vi "PC Main.vi"() -> ()   [LabVIEW 2021]
uses:
  Type Definitions/Computer Metadata.ctl
  Type Definitions/Internet Connection Monitor.ctl
  Type Definitions/CPU Usage.ctl
  Type Definitions/Disk State.ctl
  Type Definitions/Memory Monitor.ctl
  Type Definitions/System Time.ctl
  Type Definitions/Payload Class.ctl
  Type Definitions/Data Frame Header.ctl
  Type Definitions/Data Frame.ctl
  Type Definitions/Telemetry TCP State.ctl
  Type Definitions/Telemetry Recorder Status.ctl
  Type Definitions/Queue Monitor.ctl
  Type Definitions/RTOSMonitor.ctl
  Type Definitions/Enum - Commands.ctl
  Type Definitions/Command TCP State.ctl
  Type Definitions/Enum - Notification Types.ctl
  Type Definitions/Notification Data.ctl
  Type Definitions/Network Adapter State.ctl
  Type Definitions/Discovery Engine State.ctl
  Type Definitions/Digital Output Data.ctl
  Type Definitions/Analog Output Data.ctl
  <vilib>/ptbypt/NI_PtbyPt.lvlib
  Type Definitions/Computer Resources.ctl
  Type Definitions/RT Image Metadata.ctl
  Type Definitions/Startup Settings.ctl
  Type Definitions/Digital Input Data.ctl
  Type Definitions/Writeable Drives.ctl
  Type Definitions/Analog Data.ctl
  Type Definitions/GPS Solution Data.ctl
  Type Definitions/Device.ctl
  <vilib>/Utility/tcp.llb/UDP Multicast Read-Only Open.vi
  Type Definitions/Analog Output Command.ctl
  Type Definitions/Digital Output Command.ctl
panel:
  in  "Source to View":T1
  out "Data Rate (Mbps)":dbl
  out "Telemetry Rate (Packets/s)":i32
  out "Telemetry IP Address":string
  out "Detected IP Addresses":string[](array[string])
  out "Valid IP Addresses":i32
  out "Telemetry Handler":T2 {"CRC" format="%08x"; "Frame Header"."Options" format="%016b"; "Frame Header"."Time" format="%^<%I:%M:%S%3u %p\n%m/%d/%Y %Z>T"; "Frame Header"."Sync" format="%08x"}
  in  "Main Tabs":T5(tab)
  out "Computer Metadata":T6
  out "Computer Resources":T7
  out "RT Image Metadata":T8
  out "Startup Settings":T9
  out "CPU Utilization":dbl[][](graph)
  out "Available Memory":dbl[][](graph)
  out "Internet Connection Monitor":T10
  out "CPU Monitor":T11 {"Idle CPU Time" format="%#.2f"; "SIRQ CPU Usage" format="%#.2f"; "IRQ CPU Usage" format="%#.2f"; "IO CPU Usage" format="%#.2f"; "NIC CPU" format="%#.2f"; "System CPU Usage" format="%#.2f"; "User CPU Usage" format="%#.2f"}
  out "Memory Monitor":T12 {"Available Memory" format="%#.2f"; "Total Memory" format="%#.2f"}
  out "RTOS Monitor":T13[](array[typedef])
  out "Archive Monitor":T14
  out "Queue Monitor":T15[](array[typedef])
  out "System Time":T16 {"GPS Clock" format="%^<%I:%M:%S%3u %p\n%m/%d/%Y %Z>T"; "System Clock" format="%^<%I:%M:%S%3u %p\n%m/%d/%Y %Z>T"}
  out "Telemetry TCP State":T17
  out "Command TCP State":T18
  out "Network Adapter State":T19
  out "Discovery Engine State":T20[](array[typedef])
  out "Disk Management":T21[](array[typedef]) {"Used" format="%#.2f"; "Available" format="%#.2f"; "Total" format="%#.2f"}
  out "Writeable Drives":T22
  out "Digital Input Data":i16[][](graph)
  out "Analog Output Data":dbl[][](graph)
  out "Analog Input Data":sgl[][](graph)
  out "Notification Data":cluster{"Time":dbl, T23} {"Time" format="%^<%I:%M:%S%3u %p\n%m/%d/%Y %Z>T"}
  out "GPS Solution Data":T25 {"GPS Timestamp" format="%^<%I:%M:%S%3u %p\n%m/%d/%Y %Z>T"}
  in  "Send Digital Command":bool
  in  "Digital Output Command":T26
  in  "Null Command":bool
  out "Command Ack":T2 {"CRC" format="%08x"; "Frame Header"."Options" format="%016b"; "Frame Header"."Time" format="%^<%I:%M:%S%3u %p\n%m/%d/%Y %Z>T"; "Frame Header"."Sync" format="%08x"}
  out "Digital Output Data":T27 {"Port 0" format="%08b"}
  in  "Send Analog Command":bool
  in  "Analog Output Command":T28 {"State" scale=0.0..5.0}
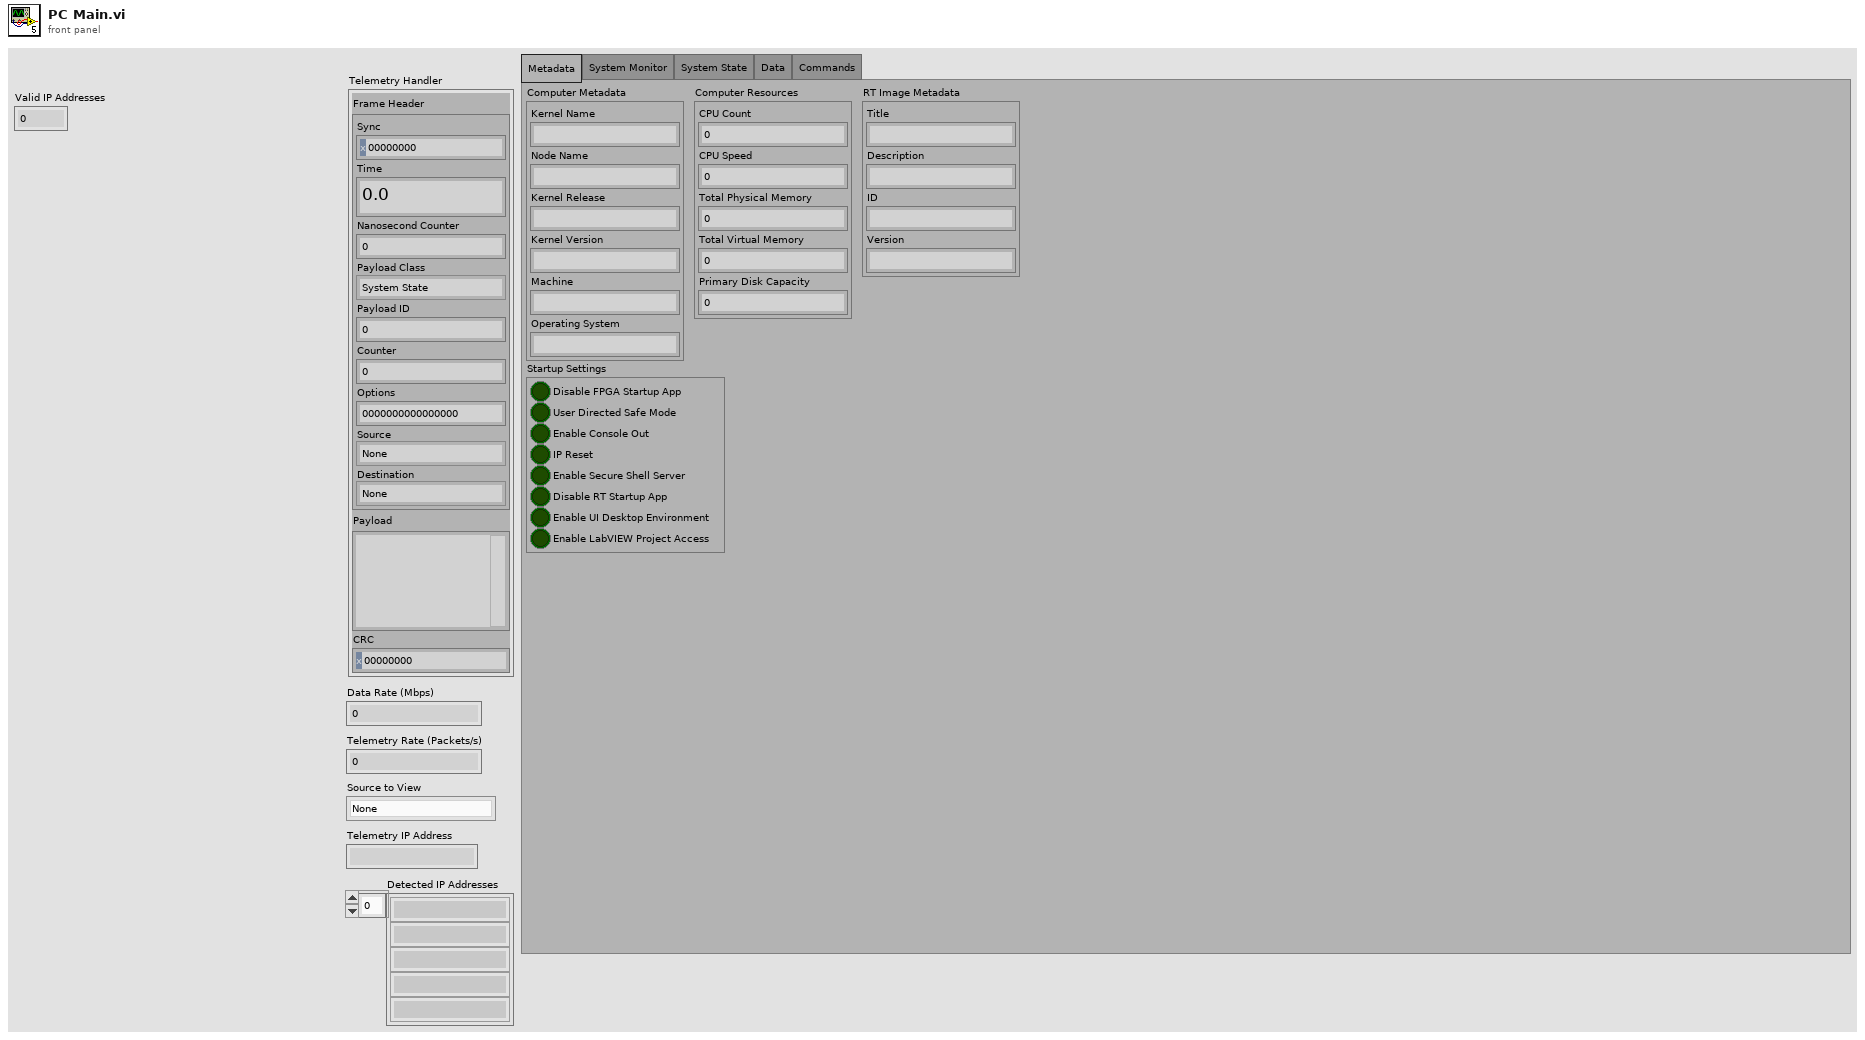
[diagram p1: front panel]
types:
  T1 = typedef "Device.ctl" = enum32{"None", "Exec", "Aux1", "Aux2", "Aux3"}
  T2 = typedef "Data Frame.ctl" = cluster{"Frame Header":T3, "Payload":string, "CRC":u32}
  T3 = typedef "Data Frame Header.ctl" = cluster{"Sync":u32, "Time":dbl, "Nanosecond Counter":i64, "Payload Class":T4, "Payload ID":u16, "Counter":i32, "Options":u32, "Source":T1, "Destination":T1}
  T4 = typedef "Payload Class.ctl" = enum16{"System State", "Parameters", "Metadata", "Software Monitor", "Data", "Commands"}
  T5 = enum32{"Metadata", "System Monitor", "System State", "Data", "Commands"}
  T6 = typedef "Computer Metadata.ctl" = cluster{"Kernel Name":string, "Node Name":string, "Kernel Release":string, "Kernel Version":string, "Machine":string, "Operating System":string}
  T7 = typedef "Computer Resources.ctl" = cluster{"CPU Count":i32, "CPU Speed":u32, "Total Physical Memory":dbl, "Total Virtual Memory":dbl, "Primary Disk Capacity":dbl}
  T8 = typedef "RT Image Metadata.ctl" = cluster{"Title":string, "Description":string, "ID":string, "Version":string}
  T9 = typedef "Startup Settings.ctl" = cluster{"Disable FPGA Startup App":bool, "User Directed Safe Mode":bool, "Enable Console Out":bool, "IP Reset":bool, "Enable Secure Shell Server":bool, "Disable RT Startup App":bool, "Enable UI Desktop Environment":bool, "Enable LabVIEW Project Access":bool}
  T10 = typedef "Internet Connection Monitor.ctl" = cluster{"Connected?":bool, "Ping Latency (uS)":i32, "Ping Address":string}
  T11 = typedef "CPU Usage.ctl" = cluster{"User CPU Usage":sgl, "System CPU Usage":sgl, "NIC CPU ":sgl, "IO CPU Usage":sgl, "IRQ CPU Usage":sgl, "SIRQ CPU Usage":sgl, "Idle CPU Time":sgl}
  T12 = typedef "Memory Monitor.ctl" = cluster{"Total Memory":sgl, "Available Memory":sgl}
  T13 = typedef "RTOSMonitor.ctl" = cluster{"Task Name":string, "Priority":i32, "Processor":i32, "Offset":i64, "Min Duration":i64, "Mean Duration":i64, "Max Duration":i64, "Period":i64, "Late Iterations":i16, "Iteration Count":i32}
  T14 = typedef "Telemetry Recorder Status.ctl" = cluster{"Filepath":string, "File Size":i64, "Frame Count":i32, "Mean MB/hour":sgl}
  T15 = typedef "Queue Monitor.ctl" = cluster{"Queue Name":string, "Max Queue Size":i32, "Pending Remove":i32, "Pending Insert":i32, "Elements in Queue":i32}
  T16 = typedef "System Time.ctl" = cluster{"System Clock":timestamp, "GPS Clock":timestamp, "Nanosecond Counter":i64, "GPS Status":enum8{"Initializing", "Normal", "Unable to get fix"}, "GPS Antenna Status":enum8{"Unknown", "Normal", "Absent", "Overcurrent"}, "GPS Satelites Available":u8, "GPS Time (ns)":u64, "GPS UTC Offset":i8, "GPS Time Offset":i32, "UTC Offset Valid":bool, "GPS Time Lock":bool}
  T17 = typedef "Telemetry TCP State.ctl" = cluster{"Is Connected":bool, "Remote Address":string, "Remote Port":u16, "Total Frames Sent":i32, "Total Bytes Sent":i32}
  T18 = typedef "Command TCP State.ctl" = cluster{"Is Connected":bool, "Remote Address":string, "Remote Port":u16, "Total Frames Sent":i32, "Total Bytes Sent":i32}
  T19 = typedef "Network Adapter State.ctl" = cluster{"Adapter IP Addresses":string[]}
  T20 = typedef "Discovery Engine State.ctl" = cluster{"Adapter IP Address":string, "Connection ID":refnum<k16>, "Error":errorcluster}
  T21 = typedef "Disk State.ctl" = cluster{"File System Name":string, "Total":sgl, "Available":sgl, "Used":sgl, "Path":string}
  T22 = typedef "Writeable Drives.ctl" = cluster{"USB/SD Drives":path[], "Hard Drives":path[]}
  T23 = typedef "Notification Data.ctl" = cluster{"Notification Type":T24, "Code":i32, "Description":string}
  T24 = typedef "Enum - Notification Types.ctl" = enum16{"Warning", "Acknowledge", "Notification"}
  T25 = typedef "GPS Solution Data.ctl" = cluster{"GPS Timestamp":timestamp, "GPS Status":enum8{"Initializing", "Normal", "Unable to get fix"}, "GPS Antenna Status":enum8{"Unknown", "Normal", "Absent", "Overcurrent"}, "GPS Satelites Available":u8, "GPS Time Lock":bool, "GPS UTC Offset Valid":bool, "GPS Self-Survey Complete":bool, "GPS Latitude (°)":dbl, "GPS Longitude (°)":dbl, "GPS Altitude (m)":dbl, "GPS Serial Number":u32, "GPS Vendor ID":u16, "GPS Firmware Version":u32}
  T26 = typedef "Digital Output Command.ctl" = cluster{"DO Channel":u8, "State":bool}
  T27 = typedef "Digital Output Data.ctl" = cluster{"Port 0":u8}
  T28 = typedef "Analog Output Command.ctl" = cluster{"AO Channel":u8, "State":dbl}
  T29 = typedef "Enum - Commands.ctl" = enum16{"Null", "Analog Output Command", "Digital Output Command"}
  T30 = typedef "Analog Data.ctl" = cluster{"Analog Data":sgl[][]}
  T31 = typedef "Analog Output Data.ctl" = cluster{"Bank 0":dbl[]}
  T32 = typedef "Digital Input Data.ctl" = cluster{"Digital Data":u64[][]}
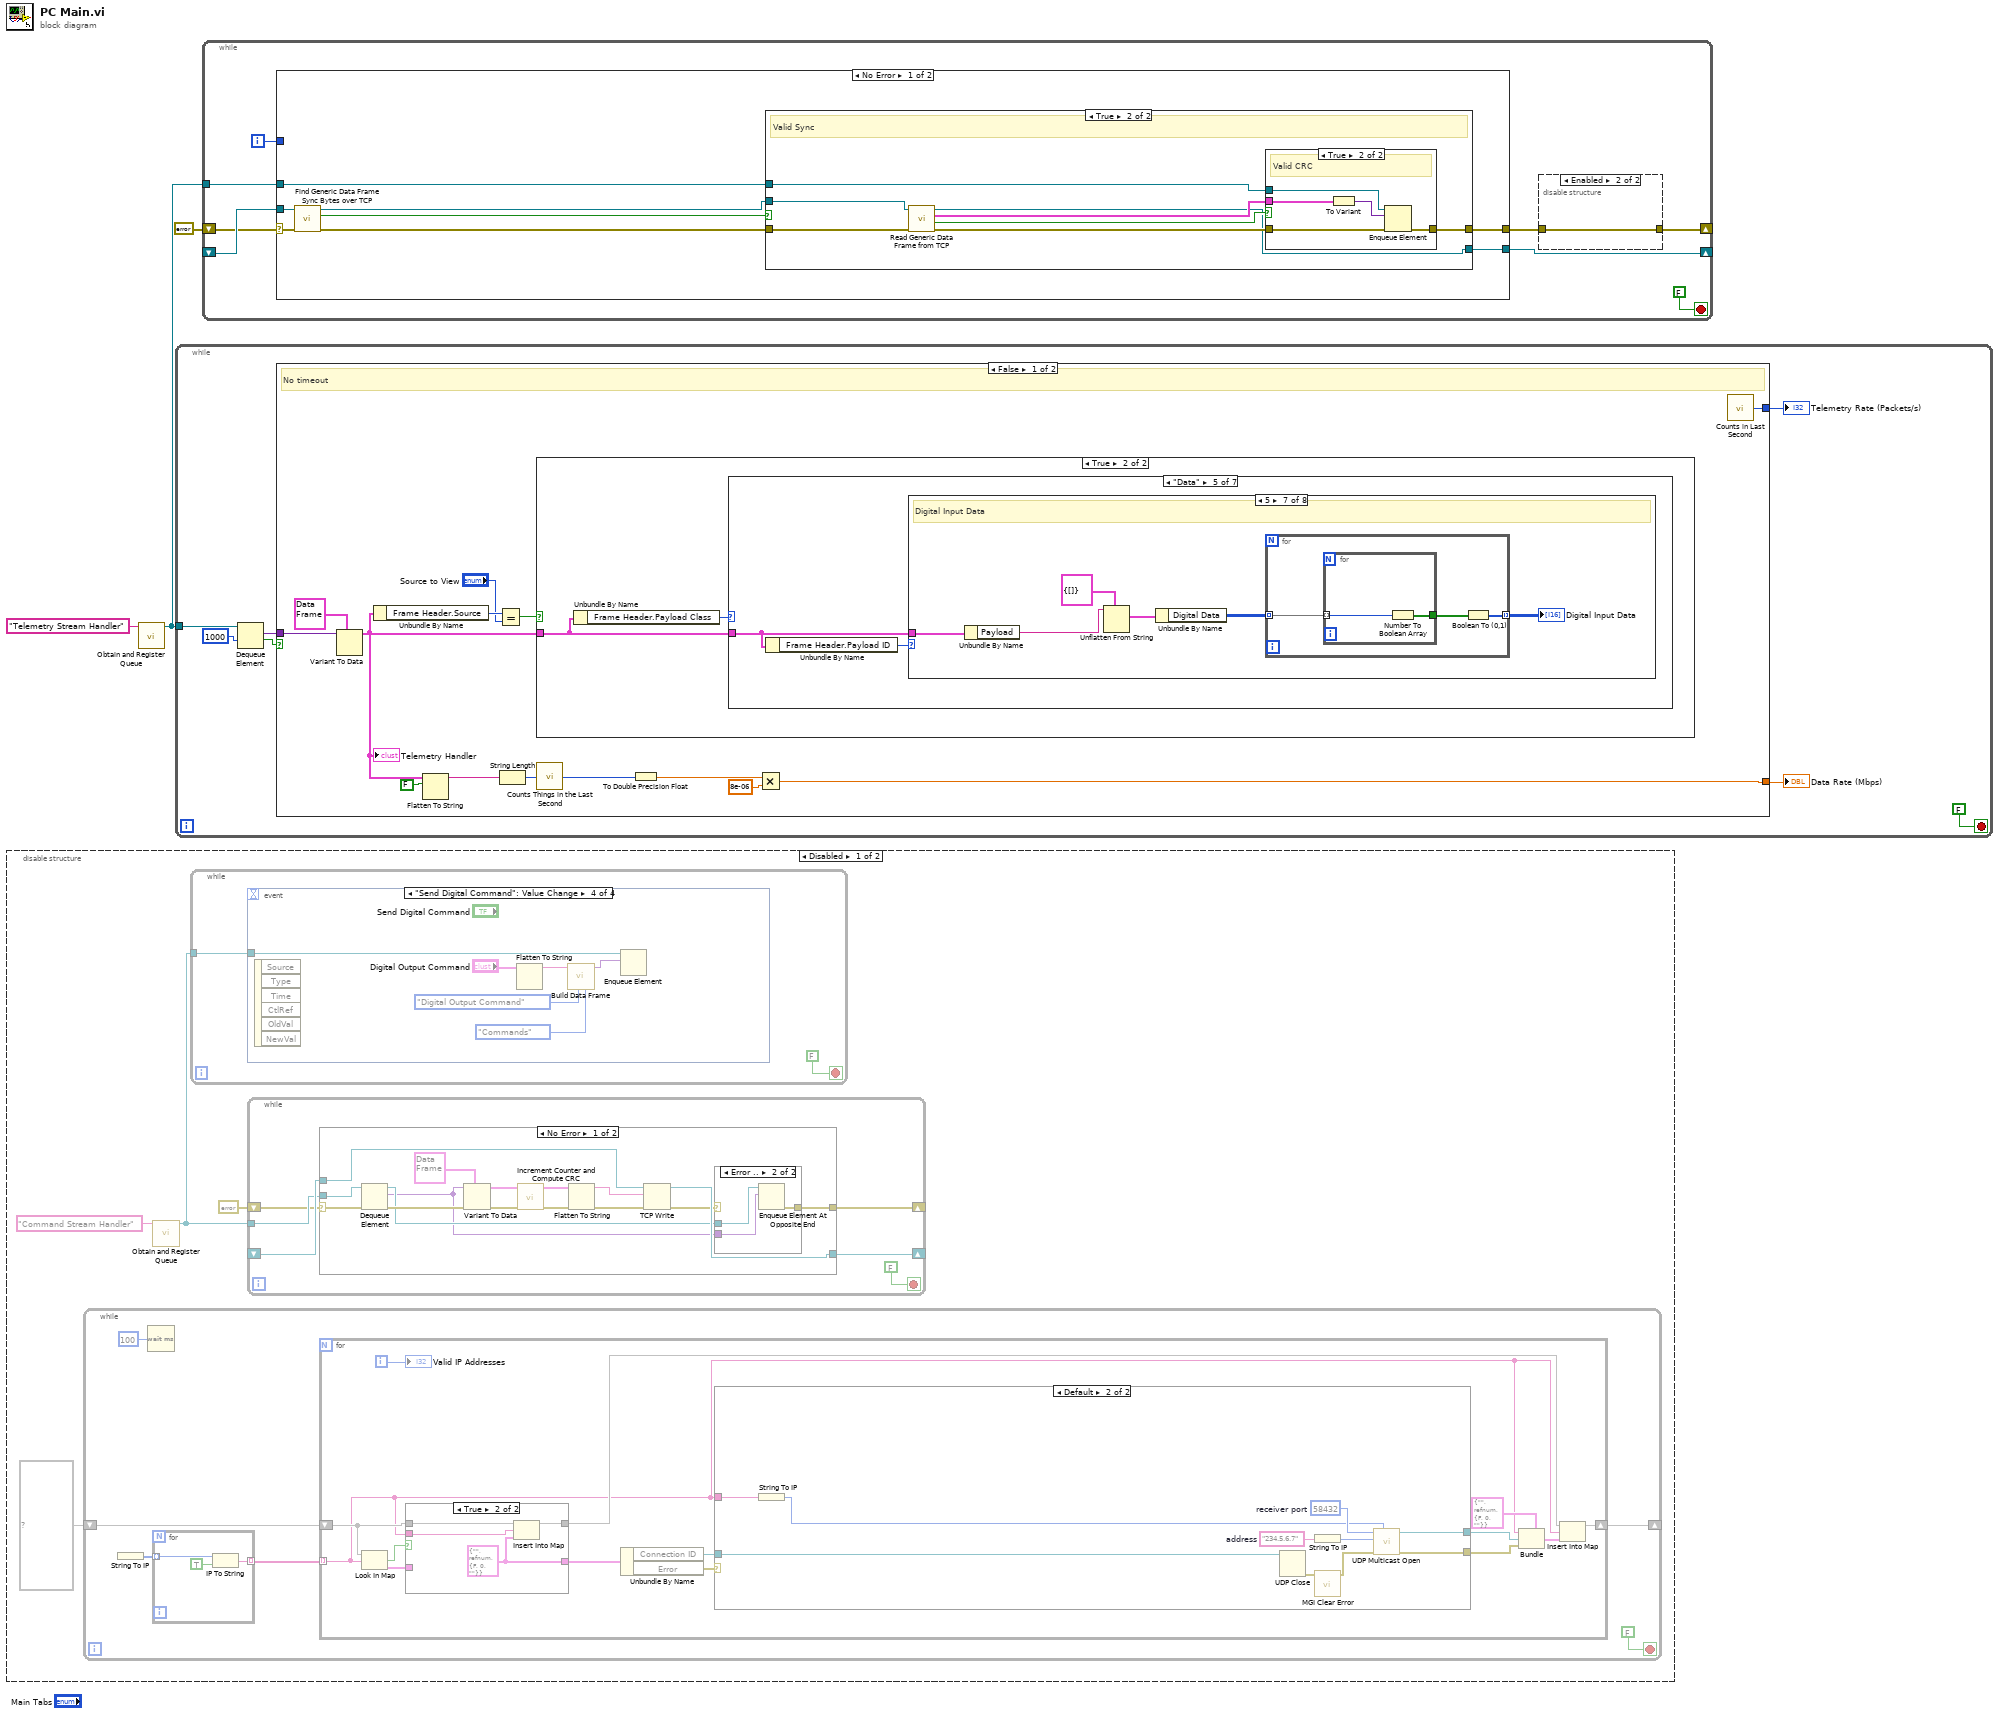
[diagram p0: block diagram]
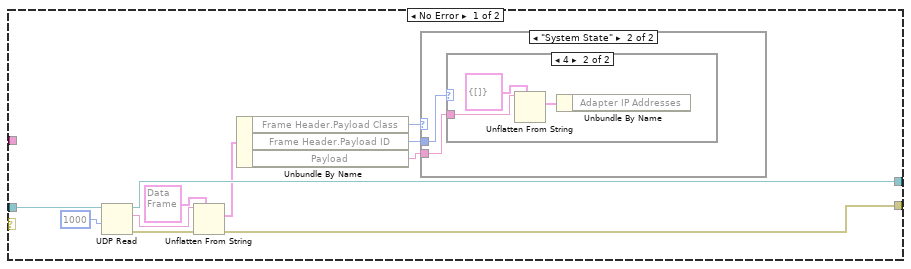
[diagram p2: hidden frame]
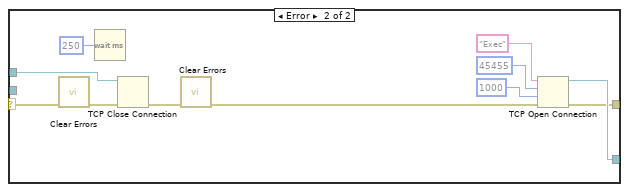
[diagram p7: hidden frame]
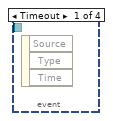
[diagram p8: hidden frame]
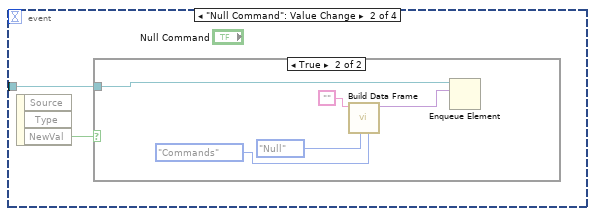
[diagram p9: hidden frame]
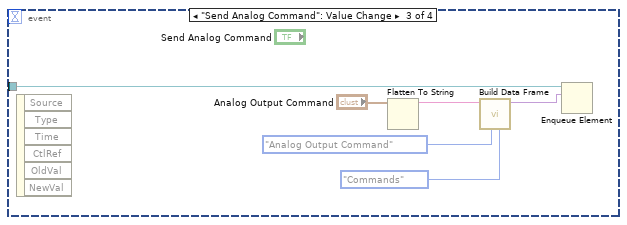
[diagram p11: hidden frame]
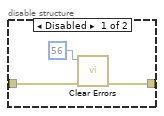
[diagram p13: hidden frame]
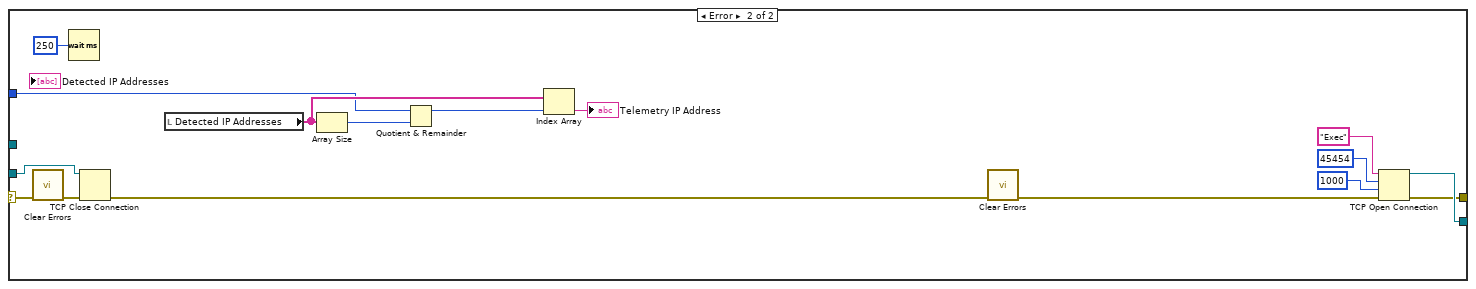
[diagram p16: hidden frame]
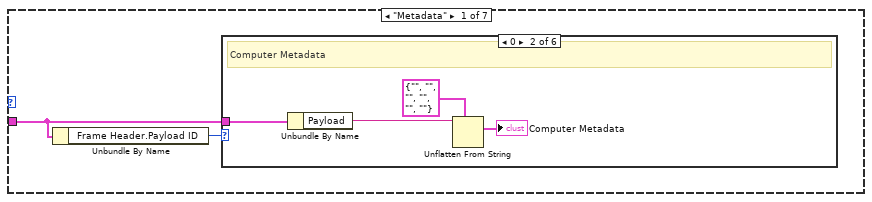
[diagram p18: hidden frame]
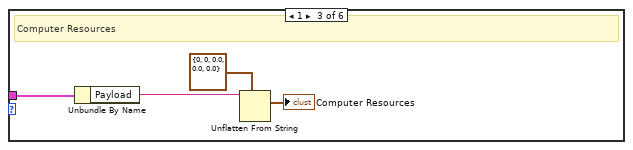
[diagram p20: hidden frame]
diagram:
  n1 = disable-structure shown="Disabled" {
    frame Disabled {
      n2 = while {
        shift-right: [w9] -> _
        shift-left: map{string, T20} {} ("map") -> [w12]
        stop <- FALSE stop-if-true
        n3 = String To IP() -> (0:w11:u32[])  [unwired: 1 in]
        n4 = Wait (ms)(milliseconds to wait=u32 100) -> ()  [unwired: 1 out]
        n5 = for {
          tunnel: w11 -> [w15] mode=indexing
          tunnel: [w14] -> w10 mode=indexing
          n6 = IP To String(1:TRUE ("dot notation? (F)"), 2:w15) -> (0:w14:string)
        }
        n7 = for {
          tunnel: w10 -> [w18] mode=indexing
          shift-right: [w17] -> w9
          shift-left: w12 -> [w29]
          i -> [w21]
          n8 = Look In Map(map=w29, key=w18) -> (key not found?=w30:bool, value=w28:T20)  [unwired: 1 in]
          n9 = case shown="True" w30 {
            tunnel: w29 -> [w58 w62]
            tunnel: w18 -> [_ w61]
            tunnel: [w58 w60] -> w24
            tunnel: w28 -> [w57 _]
            tunnel: [w57 w59] -> w27
            frame False {
            }
            frame True {
              w59 = T20 {"Adapter IP Address"="", "Connection ID"=refnum, "Error"={"status"=FALSE, "code"=0, "source"=""}} ("Connection Metadata")
              n10 = Insert Into Map(map in=w62, key=w61, value=w59) -> (map out=w60:map{string, T20})  [unwired: 2 out]
            }
          }
          n11 = Unbundle By Name(w27) -> ("Connection ID"=w26:refnum<k16>, "Error"=w25:errorcluster)
          n12 = case shown="Default" w25 {
            tunnel: [w31 w50] -> w20
            tunnel: [w39 w49] -> w19
            tunnel: w26 -> [w40 w56]
            tunnel: w18 -> [_ w55]
            frame No Error {
              n13 = UDP Read(connection ID=w40, timeout ms (25000)=1000) -> (data out=w37:string, error out=w32:errorcluster, 3:w39:refnum<k16>)  [unwired: 1 in, 3 out]
              n14 = Unflatten From String(type=T2 {"Frame Header"={"Sync"=0, "Time"=0.0, "Nanosecond Counter"=0, "Payload Class"=enum."System State", "Payload ID"=0, "Counter"=0, "Options"=0, "Source"=enum."None", "Destination"=enum."None"}, "Payload"="", "CRC"=0} ("Frame"), binary string=w37, error in (no error)=w32) -> (value=w36:T2, error out=w31:errorcluster)  [unwired: 2 in, 1 out]
              n15 = Unbundle By Name(w36) -> ("Frame Header.Payload Class"=w33:T4, "Frame Header.Payload ID"=w34:u16, "Payload"=w35:string)
              n16 = case shown="\"System State\"" w33 {
                tunnel: w35 -> [_ w43]
                tunnel: w34 -> [_ w42]
                frame Default {
                }
                frame "System State" {
                  n17 = case shown="4" w42 {
                    tunnel: w43 -> [_ w45]
                    frame 0, Default {
                    }
                    frame 4 {
                      n18 = Unflatten From String(type=T19 {"Adapter IP Addresses"=[]} ("Network Adapter Metadata"), binary string=w45) -> (value=w44:T19)  [unwired: 3 in, 2 out]
                      n19 = Unbundle By Name(w44) -> ()  [unwired: 1 out]
                    }
                  }
                }
              }
            }
            frame Default {
              w53 = u16 58432  # receiver port
              w54 = "234.5.6.7"  # address
              n20 = String To IP(1:w55) -> (0:w51:u32)
              n21 = UDP Close(connection ID=w56) -> (error out=w48:errorcluster)  [unwired: 1 in, 1 out]
              n22 = String To IP(1:w54) -> (0:w52:u32)
              n23 = call <userlib>:"MGI Clear Error.vi"("Error In"=w48) -> ("Error Out"=w47:errorcluster)  [unwired: 6 in]
              n24 = call-poly <vilib>:"UDP Multicast Open.vi"("net address"=w51, "error in (no error)"=w47, "multicast addr"=w52, "port"=w53) -> ("error out"=w50:errorcluster, "connection ID"=w49:refnum<k16>)  [unwired: 5 in, 1 out]
            }
          }
          n25 = Bundle(cluster=T20 {"Adapter IP Address"="", "Connection ID"=refnum, "Error"={"status"=FALSE, "code"=0, "source"=""}} ("Connection Metadata"), "Adapter IP Address"=w18, "Connection ID"=w19, "Error"=w20) -> (w23:T20)
          n26 = Insert Into Map(map in=w24, key=w18, value=w23) -> (map out=w17:map{string, T20})  [unwired: 2 out]
          "Valid IP Addresses" <- w21
        }
      }
      n27 = call "Obtain and Register Queue.vi"("name (unnamed)"="Command Stream Handler") -> ("Queue Out"=w6:refnum<queue>)  [unwired: 7 in, 3 out]
      n28 = while {
        tunnel: w6 -> [w100]
        stop <- FALSE stop-if-true
        n29 = event shown="[3] \"Send Digital Command\": Value Change" {
          selector: _ -> [_ _ _ _]
          dyn-events: _ -> [_ _ _ _]
          timeout: _ -> [_ _ _ _]
          tunnel: w100 -> [_ w103 w114 w120]
          event Timeout {
            n30 = event-data() -> ()  [unwired: 1 in, 3 out]
          }
          event "Null Command": Value Change {
            n31 = event-data() -> ("NewVal"=w102:bool)  [unwired: 1 in, 2 out]
            n32 = case shown="True" w102 {
              tunnel: w103 -> [_ w108]
              frame False {
              }
              frame True {
                n33 = call "Build Data Frame.vi"("Payload Class (Data)"=Payload_Class."Commands", "Payload ID (0)"=Enum_-_Commands."Null" ("Commands"), "Payload (Empty String)"="") -> ("Frame"=w107:variant)  [unwired: 7 in, 1 out]
                n34 = Enqueue Element(queue=w108, element=w107) -> ()  [unwired: 2 in, 3 out]
              }
            }
          }
          event "Send Analog Command": Value Change {
            n35 = event-data() -> ()  [unwired: 1 in, 6 out]
            n36 = Flatten To String(anything="Analog Output Command") -> (data string=w109:string)  [unwired: 3 in, 2 out]
            n37 = call "Build Data Frame.vi"("Payload Class (Data)"=Payload_Class."Commands", "Payload ID (0)"=Enum_-_Commands."Analog Output Command" ("Commands"), "Payload (Empty String)"=w109) -> ("Frame"=w112:variant)  [unwired: 7 in, 1 out]
            n38 = Enqueue Element(queue=w114, element=w112) -> ()  [unwired: 2 in, 3 out]
          }
          event "Send Digital Command": Value Change {
            n39 = event-data() -> ()  [unwired: 1 in, 6 out]
            n40 = Flatten To String(anything="Digital Output Command") -> (data string=w116:string)  [unwired: 3 in, 2 out]
            n41 = call "Build Data Frame.vi"("Payload Class (Data)"=Payload_Class."Commands", "Payload ID (0)"=Enum_-_Commands."Digital Output Command" ("Commands"), "Payload (Empty String)"=w116) -> ("Frame"=w119:variant)  [unwired: 7 in, 1 out]
            n42 = Enqueue Element(queue=w120, element=w119) -> ()  [unwired: 2 in, 3 out]
          }
        }
      }
      n43 = while {
        shift-right: [w68] -> _
        shift-left: errorcluster {"status"=TRUE, "code"=0, "source"=""} ("error out") -> [w63]
        shift-right: [w67] -> _
        shift-left: _ -> [w66]
        tunnel: w6 -> [w64]
        stop <- FALSE stop-if-true
        n44 = case shown="No Error" w63 {
          selector: w63 -> [w75 w99]
          tunnel: [w73 w92] -> w68
          tunnel: [w83 w94] -> w67
          tunnel: w66 -> [w84 w95]
          tunnel: w64 -> [w82 _]
          frame No Error {
            n45 = Dequeue Element(queue=w82, error in (no error)=w75) -> (queue out=w72:refnum<queue>, element=w71:variant, error out=w76:errorcluster)  [unwired: 1 in, 1 out]
            n46 = Variant To Data(error in=w76, type=T2 {"Frame Header"={"Sync"=0, "Time"=0.0, "Nanosecond Counter"=0, "Payload Class"=enum."System State", "Payload ID"=0, "Counter"=0, "Options"=0, "Source"=enum."None", "Destination"=enum."None"}, "Payload"="", "CRC"=0} ("Frame"), Variant=w71) -> (data=w79:T2, error out=w70:errorcluster)
            n47 = call "Increment Counter and Compute CRC.vi"("error in (no error)"=w70, "Frame In"=w79) -> ("error out"=w69:errorcluster, "Frame Out"=w78:T2)  [unwired: 8 in]
            n48 = Flatten To String(anything=w78, error in (no error)=w69) -> (data string=w80:string, error out=w77:errorcluster)  [unwired: 2 in, 1 out]
            n49 = TCP Write(connection ID=w84, data in=w80, error in (no error)=w77) -> (connection ID out=w83:refnum<k5>, error out=w74:errorcluster)  [unwired: 1 in, 1 out]
            n50 = case shown="Error .." w74 {
              selector: w74 -> [w85 _]
              tunnel: [w85 w88] -> w73
              tunnel: w72 -> [_ w87]
              tunnel: w71 -> [_ w86]
              frame No Error {
              }
              frame Error {
                n51 = Enqueue Element At Opposite End(queue=w87, element=w86) -> (error out=w88:errorcluster)  [unwired: 2 in, 2 out]
              }
            }
          }
          frame Error {
            n52 = call <vilib>:"Clear Errors.vi"("error in (no error)"=w99) -> ("error out"=w97:errorcluster)  [unwired: 5 in, 1 out]
            n53 = Wait (ms)(milliseconds to wait=u32 250) -> ()  [unwired: 1 out]
            n54 = TCP Close Connection(connection ID=w95, error in (no error)=w97) -> (error out=w96:errorcluster)  [unwired: 1 in, 1 out]
            n55 = call <vilib>:"Clear Errors.vi"("error in (no error)"=w96) -> ("error out"=w93:errorcluster)  [unwired: 5 in, 1 out]
            n56 = TCP Open Connection(address="Exec", remote port or service name=u16 45455 ("port"), timeout ms (60000)=1000 ("timeout ms (wait forever: -1)"), error in (no error)=w93) -> (connection ID=w94:refnum<k5>, error out=w92:errorcluster)  [unwired: 1 in]
          }
        }
      }
    }
    frame Enabled {
    }
  }
  n57 = call "Obtain and Register Queue.vi"("name (unnamed)"="Telemetry Stream Handler") -> ("Queue Out"=w1:refnum<queue>)  [unwired: 7 in, 3 out]
  n58 = while {
    tunnel: w1 -> [w126]
    stop <- FALSE stop-if-true
    n59 = Dequeue Element(queue=w126, timeout in ms (-1)=1000) -> (element=w127:variant, timed out?=w123:bool)  [unwired: 1 in, 2 out]
    n60 = case shown="False" w123 {
      tunnel: w127 -> [w141 _]
      tunnel: [w139 0 ("Counts In Last Second")] -> w122
      tunnel: [w132 0.0] -> w121
      frame False {
        # "No timeout"
        n61 = Variant To Data(type=T2 {"Frame Header"={"Sync"=0, "Time"=0.0, "Nanosecond Counter"=0, "Payload Class"=enum."System State", "Payload ID"=0, "Counter"=0, "Options"=0, "Source"=enum."None", "Destination"=enum."None"}, "Payload"="", "CRC"=0} ("Frame"), Variant=w141) -> (data=w131:T2)  [unwired: 1 in, 1 out]
        "Telemetry Handler" <- w131
        n62 = Unbundle By Name(w131) -> ("Frame Header.Source"=w130:T1)
        n63 = Flatten To String(anything=w131, prepend array or string size? (T)=FALSE) -> (data string=w135:string)  [unwired: 2 in, 2 out]
        n64 = Equal?(x=w130, y="Source to View") -> (x = y?=w128:bool)
        n65 = String Length(string=w135) -> (length=w136:i32)
        n66 = case shown="True" w128 {
          tunnel: w131 -> [_ w142]
          frame False {
          }
          frame True {
            n67 = Unbundle By Name(w142) -> ("Frame Header.Payload Class"=w143:T4)
            n68 = case shown="\"Data\"" w143 {
              tunnel: w142 -> [w144 w162 w165 w204 w234 _ _]
              frame "Metadata" {
                n69 = Unbundle By Name(w144) -> ("Frame Header.Payload ID"=w145:u16)
                n70 = case shown="0" w145 {
                  tunnel: w144 -> [_ w149 w153 w157 w161 _]
                  frame Default {
                  }
                  frame 0 {
                    # "Computer Metadata"
                    n71 = Unbundle By Name(w149) -> ("Payload"=w148:string)
                    n72 = Unflatten From String(type=T6 {"Kernel Name"="", "Node Name"="", "Kernel Release"="", "Kernel Version"="", "Machine"="", "Operating System"=""} ("Computer Metadata"), binary string=w148) -> (value=→"Computer Metadata":T6)  [unwired: 3 in, 2 out]
                  }
                  frame 1 {
                    # "Computer Resources"
                    n73 = Unbundle By Name(w153) -> ("Payload"=w152:string)
                    n74 = Unflatten From String(type=T7 {"CPU Count"=0, "CPU Speed"=0, "Total Physical Memory"=0.0, "Total Virtual Memory"=0.0, "Primary Disk Capacity"=0.0} ("Computer Resources"), binary string=w152) -> (value=→"Computer Resources":T7)  [unwired: 3 in, 2 out]
                  }
                  frame 2 {
                    # "RT Image Metadata"
                    n75 = Unbundle By Name(w157) -> ("Payload"=w156:string)
                    n76 = Unflatten From String(type=T8 {"Title"="", "Description"="", "ID"="", "Version"=""} ("RT Image Metadata"), binary string=w156) -> (value=→"RT Image Metadata":T8)  [unwired: 3 in, 2 out]
                  }
                  frame 3 {
                    # "Startup Settings"
                    n77 = Unbundle By Name(w161) -> ("Payload"=w160:string)
                    n78 = Unflatten From String(type=T9 {"Disable FPGA Startup App"=FALSE, "User Directed Safe Mode"=FALSE, "Enable Console Out"=FALSE, "IP Reset"=FALSE, "Enable Secure Shell Server"=FALSE, "Disable RT Startup App"=FALSE, "Enable UI Desktop Environment"=FALSE, "Enable LabVIEW Project Access"=FALSE} ("Startup Settings"), binary string=w160) -> (value=→"Startup Settings":T9)  [unwired: 3 in, 2 out]
                  }
                  frame 4 {
                    # "MOVE ME TO STATE ENUM!"
                    # "Telemetry Recorder Status"
                  }
                }
              }
              frame "Parameters" {
                n79 = Unbundle By Name(w162) -> ("Frame Header.Payload ID"=w163:u16)
                n80 = case shown="Default" w163 {
                  tunnel: w162 -> [_ _ _ _]
                  frame Default {
                  }
                  frame 0 {
                  }
                  frame 1 {
                  }
                  frame 2 {
                  }
                }
              }
              frame "Software Monitor" {
                n81 = Unbundle By Name(w165) -> ("Frame Header.Payload ID"=w164:u16)
                n82 = case shown="3" w164 {
                  tunnel: w165 -> [w169 w181 w182 w195 w196 _ w202 _]
                  frame 0 {
                    # "Internet Connection Monitor"
                    n83 = Unbundle By Name(w169) -> ("Payload"=w168:string)
                    n84 = Unflatten From String(type=T10 {"Connected?"=FALSE, "Ping Latency (uS)"=0, "Ping Address"=""} ("Internet Connection Monitor"), binary string=w168) -> (value=→"Internet Connection Monitor":T10)  [unwired: 3 in, 2 out]
                  }
                  frame 1 {
                    # "CPU Monitor"
                    n85 = Unbundle By Name(w181) -> ("Payload"=w180:string)
                    n86 = Unflatten From String(type=T11 {"User CPU Usage"=0.0, "System CPU Usage"=0.0, "NIC CPU "=0.0, "IO CPU Usage"=0.0, "IRQ CPU Usage"=0.0, "SIRQ CPU Usage"=0.0, "Idle CPU Time"=0.0}, binary string=w180) -> (value=w178:T11)  [unwired: 3 in, 2 out]
                    "CPU Monitor" <- w178
                    n87 = Unbundle By Name(w178) -> ("Idle CPU Time"=w177:sgl)
                    n88 = Subtract(x=sgl 100.0 ("y"), y=w177) -> (x-y=w173:sgl)
                    n89 = To Double Precision Float(number=w173) -> (double precision float=w172:dbl)
                    n90 = call <vilib>:"Mean PtByPt.vi"("x"=w172, "sample length"=120) -> ("mean"=w174:dbl)  [unwired: 2 in, 1 out]
                    n91 = Build Array(w174, w172) -> (w171:dbl[])
                    n92 = Build Array(w171) -> (→"CPU Utilization":dbl[][])
                  }
                  frame 2 {
                    # "Archive Monitor"
                    n93 = Unbundle By Name(w182) -> ("Payload"=w184:string)
                    n94 = Unflatten From String(type=T14 {"Filepath"="", "File Size"=0, "Frame Count"=0, "Mean MB/hour"=0.0}, binary string=w184) -> (value=→"Archive Monitor":T14)  [unwired: 3 in, 2 out]
                  }
                  frame 3 {
                    # "Memory Monitor"
                    n95 = Unbundle By Name(w195) -> ("Payload"=w194:string)
                    n96 = Unflatten From String(type=T12 {"Total Memory"=0.0, "Available Memory"=0.0}, binary string=w194) -> (value=w192:T12)  [unwired: 3 in, 2 out]
                    "Memory Monitor" <- w192
                    n97 = Unbundle By Name(w192) -> ("Available Memory"=w189:sgl)
                    n98 = To Double Precision Float(number=w189) -> (double precision float=w188:dbl)
                    n99 = call <vilib>:"Mean PtByPt.vi"("x"=w188, "sample length"=120) -> ("mean"=w190:dbl)  [unwired: 2 in, 1 out]
                    n100 = Build Array(w190, w188) -> (w187:dbl[])
                    n101 = Build Array(w187) -> (→"Available Memory":dbl[][])
                  }
                  frame 4 {
                    # "Queue Monitor"
                    n102 = Unbundle By Name(w196) -> ("Payload"=w199:string)
                    n103 = Unflatten From String(type=T15[] [] ("cluster"), binary string=w199) -> (value=→"Queue Monitor":T15[])  [unwired: 3 in, 2 out]
                  }
                  frame 5 {
                    # "RTOS Update - Not Transmitted"
                  }
                  frame 6 {
                    # "RTOS Monitor"
                    n104 = Unbundle By Name(w202) -> ("Payload"=w203:string)
                    n105 = Unflatten From String(type=T13[] [] ("cluster"), binary string=w203) -> (value=→"RTOS Monitor":T13[])  [unwired: 3 in, 2 out]
                  }
                  frame Default {
                  }
                }
              }
              frame "System State" {
                n106 = Unbundle By Name(w204) -> ("Frame Header.Payload ID"=w205:u16)
                n107 = case shown="0" w205 {
                  tunnel: w204 -> [w209 w213 w216 w221 w225 w229 w230 _]
                  frame 0 {
                    # "System Time"
                    n108 = Unbundle By Name(w209) -> ("Payload"=w208:string)
                    n109 = Unflatten From String(type=T16 {"System Clock"=timestamp(0 s since 1904-01-01), "GPS Clock"=timestamp(0 s since 1904-01-01), "Nanosecond Counter"=0, "GPS Status"=enum."Initializing", "GPS Antenna Status"=enum."Unknown", "GPS Satelites Available"=0, "GPS Time (ns)"=0, "GPS UTC Offset"=0, "GPS Time Offset"=0, "UTC Offset Valid"=FALSE, "GPS Time Lock"=FALSE}, binary string=w208) -> (value=→"System Time":T16)  [unwired: 3 in, 2 out]
                  }
                  frame 1 {
                    # "Telemetry TCP State"
                    n110 = Unbundle By Name(w213) -> ("Payload"=w212:string)
                    n111 = Unflatten From String(type=T17 {"Is Connected"=FALSE, "Remote Address"="", "Remote Port"=0, "Total Frames Sent"=0, "Total Bytes Sent"=0} ("Cluster"), binary string=w212) -> (value=→"Telemetry TCP State":T17)  [unwired: 3 in, 2 out]
                  }
                  frame 2 {
                    # "Writeable Drive State - Inactive"
                    n112 = Unbundle By Name(w216) -> ("Payload"=w217:string)
                    n113 = Unflatten From String(type=T22 {"USB/SD Drives"=[], "Hard Drives"=[]} ("Writeable Drives"), binary string=w217) -> (value=→"Writeable Drives":T22)  [unwired: 3 in, 2 out]
                  }
                  frame 3 {
                    # "Command TCP State"
                    n114 = Unbundle By Name(w221) -> ("Payload"=w220:string)
                    n115 = Unflatten From String(type=T18 {"Is Connected"=FALSE, "Remote Address"="", "Remote Port"=0, "Total Frames Sent"=0, "Total Bytes Sent"=0} ("Network Stream Status"), binary string=w220) -> (value=→"Command TCP State":T18)  [unwired: 3 in, 2 out]
                  }
                  frame 4 {
                    # "Network Adapter State"
                    n116 = Unbundle By Name(w225) -> ("Payload"=w224:string)
                    n117 = Unflatten From String(type=T19 {"Adapter IP Addresses"=[]}, binary string=w224) -> (value=→"Network Adapter State":T19)  [unwired: 3 in, 2 out]
                  }
                  frame 5 {
                    # "Discovery Engine State"
                    n118 = Unbundle By Name(w229) -> ("Payload"=w228:string)
                    n119 = Unflatten From String(type=T20[] [] ("Array"), binary string=w228) -> (value=→"Discovery Engine State":T20[])  [unwired: 3 in, 2 out]
                  }
                  frame 6 {
                    # "Disk State"
                    n120 = Unbundle By Name(w230) -> ("Payload"=w233:string)
                    n121 = Unflatten From String(type=T21[] [], binary string=w233) -> (value=→"Disk Management":T21[])  [unwired: 3 in, 2 out]
                  }
                  frame Default {
                  }
                }
              }
              frame "Data" {
                n122 = Unbundle By Name(w234) -> ("Frame Header.Payload ID"=w235:u16)
                n123 = case shown="5" w235 {
                  tunnel: w234 -> [_ w240 w246 w252 w256 w260 w266 w275]
                  frame Default {
                  }
                  frame 0 {
                    # "Analog Input Data"
                    n124 = Unbundle By Name(w240) -> ("Payload"=w239:string)
                    n125 = Unflatten From String(type=T30 {"Analog Data"=[]} ("Analog Data"), binary string=w239) -> (value=w238:T30)  [unwired: 3 in, 2 out]
                    n126 = Unbundle By Name(w238) -> ("Analog Data"=→"Analog Input Data":sgl[][])
                  }
                  frame 1 {
                    # "Notification Data"
                    n127 = Unbundle By Name(w246) -> ("Frame Header.Time"=w243:dbl, "Payload"=w245:string)
                    n128 = Unflatten From String(type=T23 {"Notification Type"=enum."Warning", "Code"=0, "Description"=""}, binary string=w245) -> (value=w242:T23)  [unwired: 3 in, 2 out]
                    n129 = Bundle("Time"=w243, w242) -> (→"Notification Data":cluster{"Time":dbl, T23})  [unwired: 1 in]
                  }
                  frame 2 {
                    # "Analog Output Data"
                    n130 = Unbundle By Name(w252) -> ("Payload"=w251:string)
                    n131 = Unflatten From String(type=T31 {"Bank 0"=[]}, binary string=w251) -> (value=w248:T31)  [unwired: 3 in, 2 out]
                    n132 = Unbundle By Name(w248) -> ("Bank 0"=w247:dbl[])
                    n133 = Build Array(w247) -> (→"Analog Output Data":dbl[][])
                  }
                  frame 3 {
                    # "Digital Output Data"
                    n134 = Unbundle By Name(w256) -> ("Payload"=w255:string)
                    n135 = Unflatten From String(type=T27 {"Port 0"=0}, binary string=w255) -> (value=→"Digital Output Data":T27)  [unwired: 3 in, 2 out]
                  }
                  frame 4 {
                    # "Command Ack"
                    n136 = Unbundle By Name(w260) -> ("Payload"=w259:string)
                    n137 = Unflatten From String(type=T2 {"Frame Header"={"Sync"=0, "Time"=0.0, "Nanosecond Counter"=0, "Payload Class"=enum."System State", "Payload ID"=0, "Counter"=0, "Options"=0, "Source"=enum."None", "Destination"=enum."None"}, "Payload"="", "CRC"=0} ("Frame"), binary string=w259) -> (value=→"Command Ack":T2)  [unwired: 3 in, 2 out]
                  }
                  frame 5 {
                    # "Digital Input Data"
                    n138 = Unbundle By Name(w266) -> ("Payload"=w265:string)
                    n139 = Unflatten From String(type=T32 {"Digital Data"=[]} ("Digital Input Data"), binary string=w265) -> (value=w264:T32)  [unwired: 3 in, 2 out]
                    n140 = Unbundle By Name(w264) -> ("Digital Data"=w263:u64[][])
                    n141 = for {
                      tunnel: w263 -> [w269] mode=indexing
                      tunnel: [w267] -> w262 mode=indexing
                      n142 = for {
                        tunnel: w269 -> [w271] mode=indexing
                        tunnel: [w270] -> w268
                        n143 = Number To Boolean Array(number=w271) -> (Boolean array=w270:bool[])
                      }
                      n144 = Boolean To (0,1)(Boolean=w268) -> (0, 1=w267:i16[])
                    }
                    "Digital Input Data" <- w262
                  }
                  frame 6 {
                    # "GPS Solution Data"
                    n145 = Unbundle By Name(w275) -> ("Payload"=w274:string)
                    n146 = Unflatten From String(type=T25 {"GPS Timestamp"=timestamp(0 s since 1904-01-01), "GPS Status"=enum."Initializing", "GPS Antenna Status"=enum."Unknown", "GPS Satelites Available"=0, "GPS Time Lock"=FALSE, "GPS UTC Offset Valid"=FALSE, "GPS Self-Survey Complete"=FALSE, "GPS Latitude (°)"=0.0, "GPS Longitude (°)"=0.0, "GPS Altitude (m)"=0.0, "GPS Serial Number"=0, "GPS Vendor ID"=0, "GPS Firmware Version"=0} ("GPS Solution Data"), binary string=w274) -> (value=→"GPS Solution Data":T25)  [unwired: 3 in, 2 out]
                  }
                }
              }
              frame "Commands" {
              }
              frame Default {
              }
            }
          }
        }
        n147 = call "Counts Things in the Last Second.vi"("Things to Count"=w136) -> ("Counts In Last Second"=w137:i32)  [unwired: 4 in]
        n148 = To Double Precision Float(number=w137) -> (double precision float=w138:dbl)
        n149 = Multiply(x=w138, y=8e-06) -> (x*y=w132:dbl)
        n150 = call "Counts in Last Second.vi"() -> ("Counts In Last Second"=w139:i32)  [unwired: 5 in]
      }
      frame True {
      }
    }
    "Telemetry Rate (Packets/s)" <- w122
    "Data Rate (Mbps)" <- w121
  }
  n151 = while {
    shift-right: [w278] -> _
    shift-left: errorcluster {"status"=TRUE, "code"=0, "source"=""} ("error in (no error)") -> [w281]
    shift-right: [w285] -> _
    shift-left: _ -> [w284]
    tunnel: w1 -> [w282]
    i -> [w280]
    stop <- FALSE stop-if-true
    n152 = case shown="No Error" w281 {
      selector: w281 -> [w297 w329]
      tunnel: [w292 w322] -> w279
      tunnel: [w294 w324] -> w285
      tunnel: w284 -> [w296 w325]
      tunnel: w282 -> [w290 _]
      tunnel: w280 -> [_ w315]
      frame No Error {
        n153 = call "Find Generic Data Frame Sync Bytes over TCP.vi"("error in (no error)"=w297, "TCP Network Connection in"=w296) -> ("error out"=w293:errorcluster, "Valid Sync"=w291:bool, "TCP Network Connection out"=w295:refnum<k5>)  [unwired: 7 in]
        n154 = case shown="True" w291 {
          tunnel: w295 -> [w299 w307]
          tunnel: [w299 w300] -> w294
          tunnel: w293 -> [w298 w306]
          tunnel: [w298 w301] -> w292
          tunnel: w290 -> [_ w303]
          frame False {
            # "Invalid Sync"
          }
          frame True {
            # "Valid Sync"
            n155 = call "Read Generic Data Frame from TCP.vi"("error in (no error)"=w306, "TCP Network Connection in"=w307) -> ("error out"=w302:errorcluster, "Valid CRC"=w304:bool, "Frame Received"=w305:T2, "TCP Network Connection out"=w300:refnum<k5>)  [unwired: 6 in]
            n156 = case shown="True" w304 {
              tunnel: w305 -> [_ w309]
              tunnel: w303 -> [_ w313]
              tunnel: w302 -> [w308 w312]
              tunnel: [w308 w311] -> w301
              frame False {
                # "Invalid CRC"
              }
              frame True {
                # "Valid CRC"
                n157 = To Variant(anything=w309) -> (Variant=w310:variant)
                n158 = Enqueue Element(queue=w313, element=w310, error in (no error)=w312) -> (error out=w311:errorcluster)  [unwired: 1 in, 2 out]
              }
            }
          }
        }
      }
      frame Error {
        n159 = call <vilib>:"Clear Errors.vi"("error in (no error)"=w329) -> ("error out"=w327:errorcluster)  [unwired: 5 in, 1 out]
        n160 = Wait (ms)(milliseconds to wait=u32 250) -> ()  [unwired: 1 out]
        n161 = TCP Close Connection(connection ID=w325, error in (no error)=w327) -> (error out=w326:errorcluster)  [unwired: 1 in, 1 out]
        n162 = local read "Detected IP Addresses"() -> (w317:string[])
        n163 = Array Size(array=w317) -> (size(s)=w318:i32)
        n164 = Quotient & Remainder(x=w315, y=w318) -> (x-y*floor(x/y)=w319:i32)  [unwired: 1 out]
        n165 = Index Array(array=w317, index=w319) -> (element=→"Telemetry IP Address":string)
        n166 = call <vilib>:"Clear Errors.vi"("error in (no error)"=w326) -> ("error out"=w323:errorcluster)  [unwired: 5 in, 1 out]
        n167 = TCP Open Connection(address="Exec", remote port or service name=u16 45454 ("port"), timeout ms (60000)=1000 ("timeout ms (wait forever: -1)"), error in (no error)=w323) -> (connection ID=w324:refnum<k5>, error out=w322:errorcluster)  [unwired: 1 in]
      }
    }
    n168 = disable-structure shown="Enabled" {
      disable-tunnel: w279 -> [w287 w289]
      disable-tunnel: [w286 w289] -> w278
      frame Disabled {
        n169 = call <vilib>:"Clear Errors.vi"("error in (no error)"=w287, "specific error code to clear (0: all)"=56) -> ("error out"=w286:errorcluster)  [unwired: 4 in, 1 out]
      }
      frame Enabled {
      }
    }
  }
